vi "Decode Publish Package (Raw).vi"(8 "error in (no error)":errorcluster, 10 "PUBLISH in":refnum<class "PUBLISH.lvclass">, 11 "MQTT_Base in":refnum<class "MQTT_Base.lvclass">) -> (0 "error out":errorcluster, 1 "Payload":u8[](array[numeric]) format="%08b", 2 "Topic":string, 3 "MQTT_Base out":refnum<class "MQTT_Base.lvclass">)   [LabVIEW 2013, in "MQTT Server.lvlib" / "MQTT_Base.lvclass"]
uses:
  MQTT_Base.lvclass
  Control Packets/PUBLISH/PUBLISH.lvclass
  Control Packets/ControlPacket/ControlPacket.lvclass/ControlPacket.ctl
  Control Packets/ControlPacket/ControlPacket.lvclass
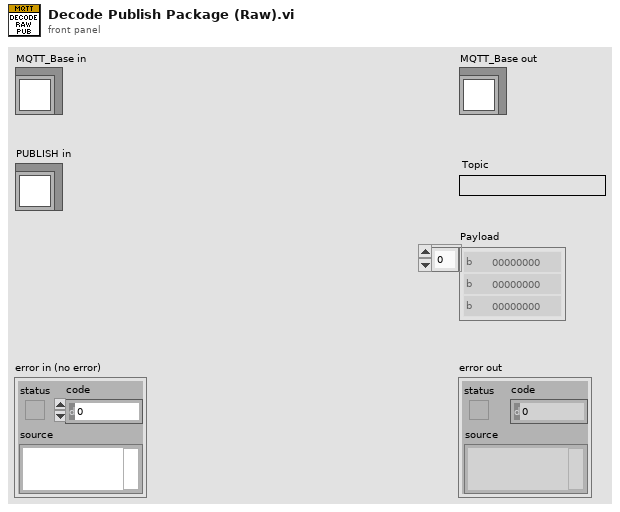
[diagram p1: front panel]
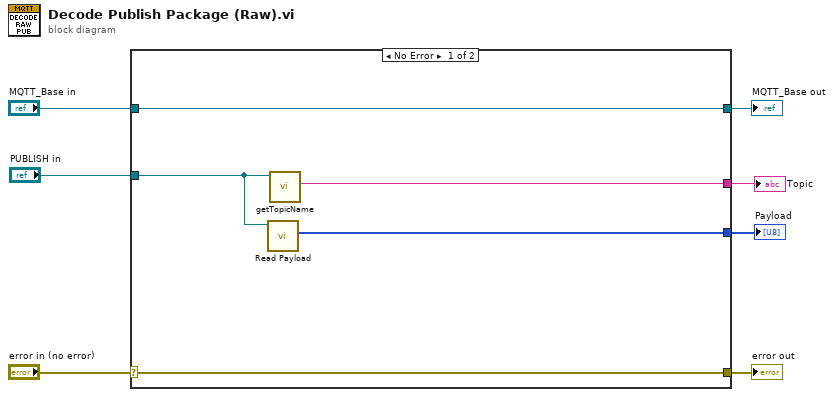
[diagram p0: block diagram]
diagram:
  n1 = case shown="No Error" "error in (no error)" {
    selector: "error in (no error)" -> [w8 w14]
    tunnel: [w8 w14] -> w6
    tunnel: [w12 w13] -> w4
    tunnel: "MQTT_Base in" -> [w12 w13]
    tunnel: "PUBLISH in" -> [w10 _]
    tunnel: [w11 _] -> w2
    tunnel: [w9 _] -> w1
    frame No Error {
      n2 = call "Read Payload.vi"("ControlPacket in"=w10) -> ("Payload"=w9:u8[])  [unwired: 9 in, 1 out]
      n3 = call "getTopicName.vi"("PUBLISH in"=w10) -> ("Topic"=w11:string)  [unwired: 8 in, 2 out]
    }
    frame Error {
    }
  }
  "error out" <- w6
  "MQTT_Base out" <- w4
  "Topic" <- w2
  "Payload" <- w1
